vi "Tool sub node list.vi"(7 "Tool node":u8, 11 "error in (no error)":errorcluster) -> (2 "Main node address":u8, 3 "Via master":bool, 4 "LEIN Variation":T2, 8 "SID":u8, 10 "Exp len":T1={"LEIN 0(error)"=7, "LEIN 1(Task)"=7, "LEIN 2(stat2)"=60, "LEIN 14(Debug)"=60, "LEIN 15(ID)"=10}, 13 "node registered":bool, 14 "Node name":string, 15 "error out":errorcluster)   [LabVIEW 2011]
uses:
  LEINmaster/Defenitions/LEIN Structure variations.ctl
  LEINmaster/Defenitions/Expected STAT lenght cluster.ctl
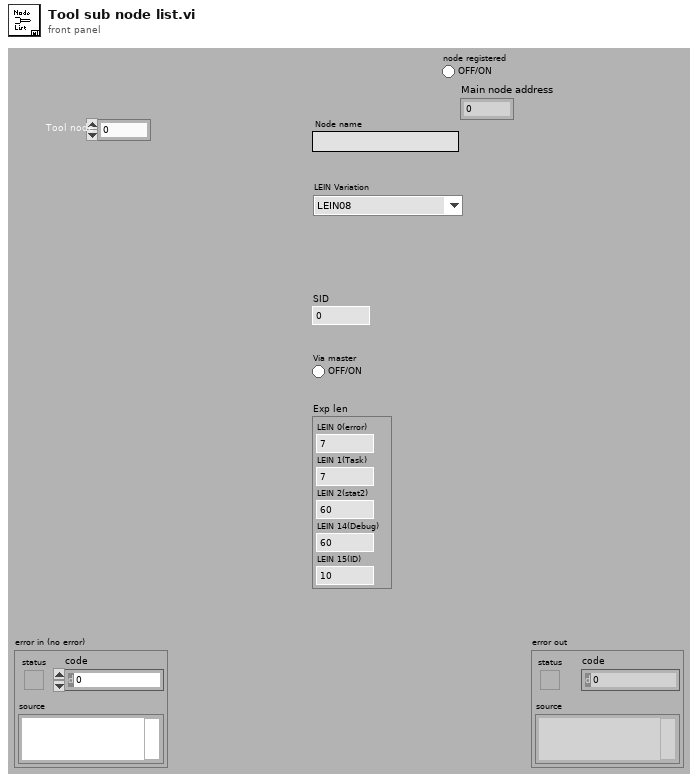
[diagram p1: front panel]
types:
  T1 = typedef "Expected STAT lenght cluster.ctl" = cluster{"LEIN 0(error)":u16, "LEIN 1(Task)":u16, "LEIN 2(stat2)":u16, "LEIN 14(Debug)":u16, "LEIN 15(ID)":u16}
  T2 = typedef "LEIN Structure variations.ctl" = enum16{"LEIN08", "LEIN31", "LEIN63"}
  T3 = typedef "List of tools.ctl" = enum16{"Stroker", "Driller", "Tractor"}
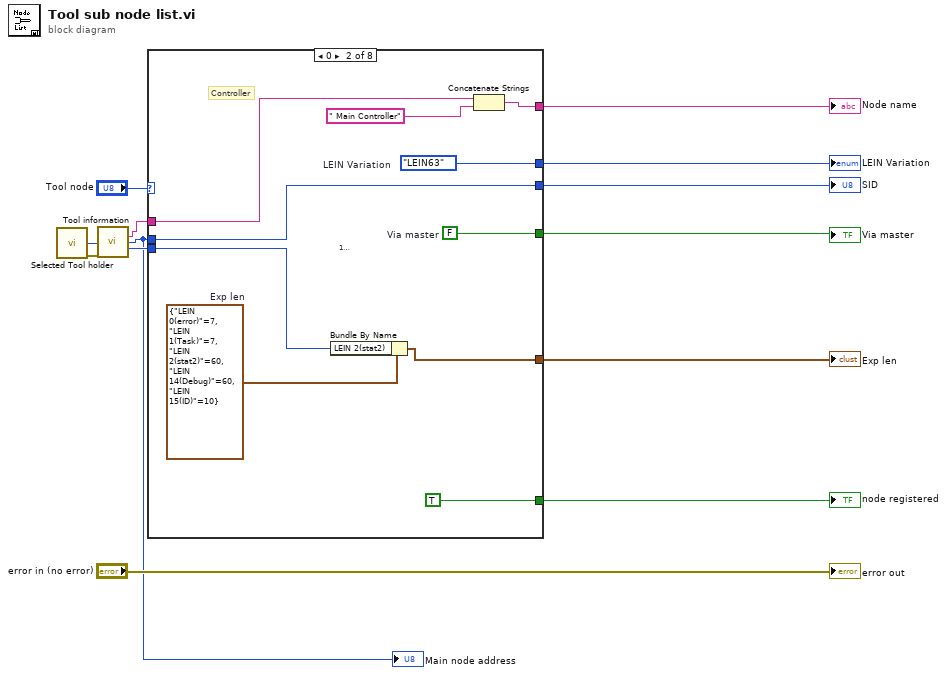
[diagram p0: block diagram]
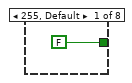
[diagram p2: hidden frame]
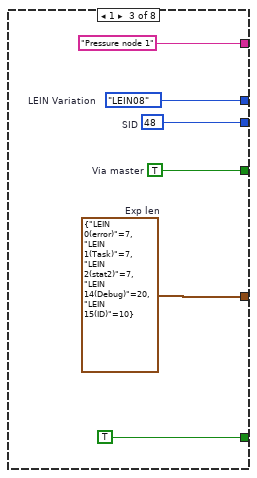
[diagram p3: hidden frame]
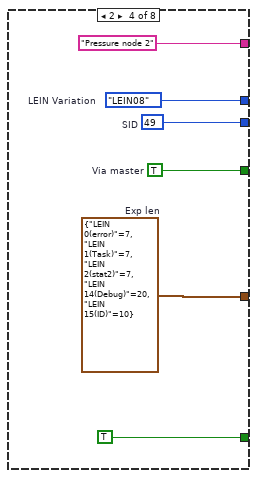
[diagram p4: hidden frame]
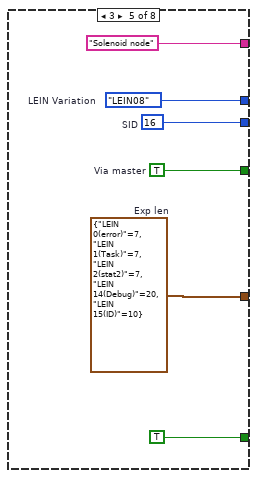
[diagram p5: hidden frame]
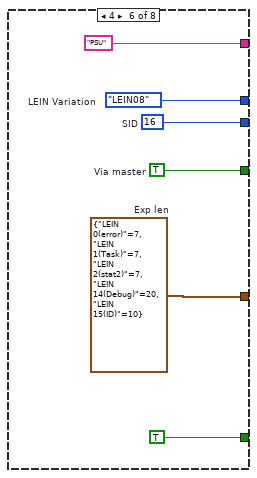
[diagram p6: hidden frame]
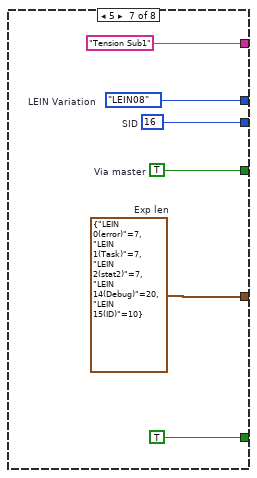
[diagram p7: hidden frame]
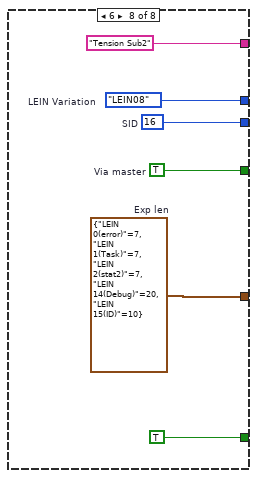
[diagram p8: hidden frame]
diagram:
  n1 = call "Selected Tool holder.vi"() -> ("Tool out"=w5:T3, "error out"=w4:errorcluster)  [unwired: 14 in]
  n2 = call "Tool information.vi"("Tool in"=w5, "error in (no error)"=w4) -> ("Tool (folder) name"=w1:string, "Main node address"=w2:u8, "Expected stat 2 message len"=w3:u8)  [unwired: 10 in, 1 out]
  "Main node address" <- w2
  n3 = case shown="0" "Tool node" {
    tunnel: [_ w24 w30 w36 w42 w48 w54 w60] -> w9
    tunnel: [_ w16 w29 w35 w41 w47 w53 w59] -> w10
    tunnel: [_ w23 w28 w34 w40 w46 w52 w58] -> w12
    tunnel: [_ w20 w27 w33 w39 w45 w51 w57] -> w13
    tunnel: [_ w18 "Pressure node 1" "Pressure node 2" "Solenoid node" "PSU" "Tension Sub1" "Tension Sub2"] -> w11
    tunnel: [FALSE TRUE TRUE TRUE TRUE TRUE TRUE TRUE] -> w7
    tunnel: w3 -> [_ w17 _ _ _ _ _ _]
    tunnel: w2 -> [_ w16 _ _ _ _ _ _]
    tunnel: w1 -> [_ w15 _ _ _ _ _ _]
    frame 255, Default {
    }
    frame 0 {
      w19 = T1 {"LEIN 0(error)"=7, "LEIN 1(Task)"=7, "LEIN 2(stat2)"=60, "LEIN 14(Debug)"=60, "LEIN 15(ID)"=10}  # Exp len
      w23 = FALSE  # Via master
      w24 = LEIN_Structure_variations."LEIN63"  # LEIN Variation
      # "1.3"
      # "Controller"
      n4 = Bundle By Name(cluster=w19, "LEIN 2(stat2)"=w17) -> (w20:T1)
      n5 = Concatenate Strings(w15, " Main Controller") -> (w18:string)
    }
    frame 1 {
      w27 = T1 {"LEIN 0(error)"=7, "LEIN 1(Task)"=7, "LEIN 2(stat2)"=7, "LEIN 14(Debug)"=20, "LEIN 15(ID)"=10}  # Exp len
      w28 = TRUE  # Via master
      w29 = u8 48  # SID
      w30 = LEIN_Structure_variations."LEIN08"  # LEIN Variation
    }
    frame 2 {
      w33 = T1 {"LEIN 0(error)"=7, "LEIN 1(Task)"=7, "LEIN 2(stat2)"=7, "LEIN 14(Debug)"=20, "LEIN 15(ID)"=10}  # Exp len
      w34 = TRUE  # Via master
      w35 = u8 49  # SID
      w36 = LEIN_Structure_variations."LEIN08"  # LEIN Variation
    }
    frame 3 {
      w39 = T1 {"LEIN 0(error)"=7, "LEIN 1(Task)"=7, "LEIN 2(stat2)"=7, "LEIN 14(Debug)"=20, "LEIN 15(ID)"=10}  # Exp len
      w40 = TRUE  # Via master
      w41 = u8 16  # SID
      w42 = LEIN_Structure_variations."LEIN08"  # LEIN Variation
    }
    frame 4 {
      w45 = T1 {"LEIN 0(error)"=7, "LEIN 1(Task)"=7, "LEIN 2(stat2)"=7, "LEIN 14(Debug)"=20, "LEIN 15(ID)"=10}  # Exp len
      w46 = TRUE  # Via master
      w47 = u8 16  # SID
      w48 = LEIN_Structure_variations."LEIN08"  # LEIN Variation
    }
    frame 5 {
      w51 = T1 {"LEIN 0(error)"=7, "LEIN 1(Task)"=7, "LEIN 2(stat2)"=7, "LEIN 14(Debug)"=20, "LEIN 15(ID)"=10}  # Exp len
      w52 = TRUE  # Via master
      w53 = u8 16  # SID
      w54 = LEIN_Structure_variations."LEIN08"  # LEIN Variation
    }
    frame 6 {
      w57 = T1 {"LEIN 0(error)"=7, "LEIN 1(Task)"=7, "LEIN 2(stat2)"=7, "LEIN 14(Debug)"=20, "LEIN 15(ID)"=10}  # Exp len
      w58 = TRUE  # Via master
      w59 = u8 16  # SID
      w60 = LEIN_Structure_variations."LEIN08"  # LEIN Variation
    }
  }
  "LEIN Variation" <- w9
  "SID" <- w10
  "Node name" <- w11
  "Via master" <- w12
  "Exp len" <- w13
  "node registered" <- w7
  "error out" <- "error in (no error)"
